vi "Command_Flywheel_SpinUp.vi"(7 "Startup":bool, 9 "Timeout":dbl, 10 "Speed":dbl) -> (2 "Flywheel_Output":dbl, 4 "Reint":bool, 6 "Completed":bool)   [LabVIEW 2020]
uses:
  Auto Utilities/Command_Execution_State.ctl
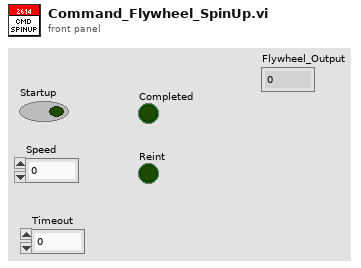
[diagram p1: front panel]
types:
  T1 = typedef "Command_Execution_State.ctl" = enum16{"Initialize", "Execute", "Finish"}
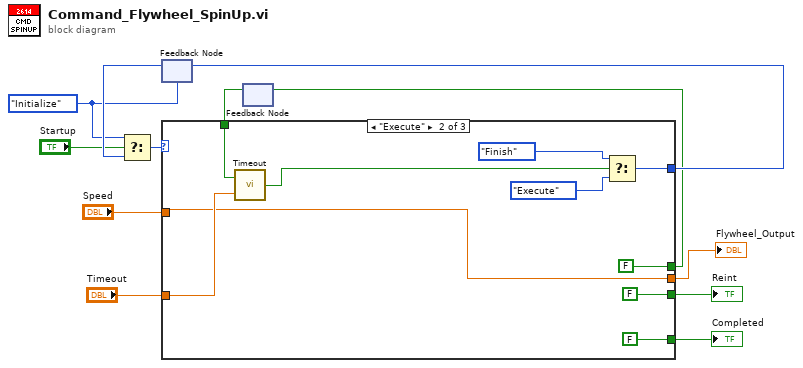
[diagram p0: block diagram]
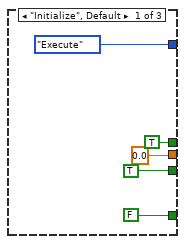
[diagram p2: hidden frame]
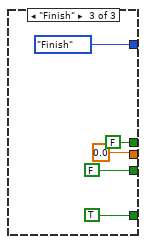
[diagram p3: hidden frame]
diagram:
  w6 = Command_Execution_State."Initialize" ("Play State")
  n1 = feedback #1(w6) -> (w10:T1)
  n2 = Select(t=w6, s="Startup", f=w10) -> (s? t:f=w12:T1)
  n3 = feedback #2() -> (w4:bool)  [unwired: 1 in]
  n4 = case shown="\"Execute\"" w12 {
    tunnel: [Command_Execution_State."Execute" ("Play State") w21 Command_Execution_State."Finish" ("Play State")] -> w11
    tunnel: [FALSE FALSE TRUE] -> w9
    tunnel: [TRUE FALSE FALSE] -> w7
    tunnel: [TRUE FALSE FALSE] -> w5
    tunnel: w4 -> [_ w24 _]
    tunnel: "Timeout" -> [_ w23 _]
    tunnel: [0.0 ("Speed") w22 0.0 ("Speed")] -> w2
    tunnel: "Speed" -> [_ w22 _]
    frame "Initialize", Default {
    }
    frame "Execute" {
      n5 = call "Timeout.vi"("Timeout"=w23, "Initialize"=w24) -> ("Timed Out?"=w18:bool)
      n6 = Select(t=Command_Execution_State."Finish" ("Play State"), s=w18, f=Command_Execution_State."Execute" ("Play State")) -> (s? t:f=w21:T1)
    }
    frame "Finish" {
    }
  }
  "Completed" <- w9
  "Reint" <- w7
  "Flywheel_Output" <- w2
  n7 = feedback-in #1(w11) -> ()
  n8 = feedback-in #2(w5) -> ()
